vi "hamamatsuSetExternalTrigger.vi"   [LabVIEW 2017]
uses:
  globalDevices.vi
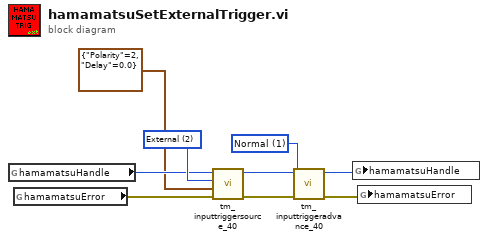
[diagram p0: block diagram]
diagram:
  w3 = 1 items=["Normal"=1, "PIV"=3, "Start Trigger"=6, "Multigate"=7, "Multiframe"=8] ("option")
  w9 = 2 items=["Internal"=1, "External"=2, "Software"=3, "Master Pulse"=4] ("Source")
  n1 = global read "globalDevices.vi" "hamamatsuHandle"() -> (w7:u32)
  n2 = global read "globalDevices.vi" "hamamatsuError"() -> (w8:errorcluster)
  n3 = call <userlib>:"tm_inputtriggersource_40.vi"("error in (no error)"=w8, "External Options"=cluster{"Polarity":i32, "Delay":dbl} {"Polarity"=2, "Delay"=0.0}, "Source"=w9, "Handle in"=w7) -> ("error out"=w4:errorcluster, "Handle out"=w5:u32)  [unwired: 6 in]
  n4 = call <userlib>:"tm_inputtriggeradvance_40.vi"("error in (no error)"=w4, "option"=w3, "Handle in"=w5) -> ("error out"=w1:errorcluster, "Handle out"=w2:u32)  [unwired: 7 in]
  n5 = global write "globalDevices.vi" "hamamatsuHandle"(w2) -> ()
  n6 = global write "globalDevices.vi" "hamamatsuError"(w1) -> ()
